vi "Initialize LMS Filter.vi"(0 "reference in":refnum<class "AdvSigProc.lvclass">, 5 "error in (no error)":errorcluster, 6 "Reset Filter?":bool=TRUE) -> (14 "reference out":refnum<class "AdvSigProc.lvclass">, 19 "error out":errorcluster)   [LabVIEW 2020, in "AdvSigProc.lvclass"]
uses:
  AdvSigProc.lvclass
  protected/Iteration Metrics.ctl
  <vilib>/addons/Adaptive Filters/Create/AFT Create FIR LMS (Real).vi
  <vilib>/addons/Adaptive Filters/Create/AFT Create FIR RLS (Real).vi
  <vilib>/addons/Adaptive Filters/Create/AFT Create FIR QR-RLS (Real).vi
  <vilib>/addons/Adaptive Filters/Create/AFT Create FIR Normalized LMS (Real).vi
  <vilib>/addons/Adaptive Filters/NI_AdaptiveFilter.lvlib
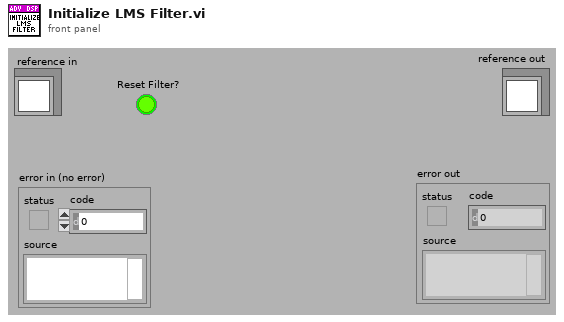
[diagram p1: front panel]
types:
  T1 = typedef "AdvSigProc.lvclass/Iteration Metrics.ctl" = cluster{"Name":string, "Max":dbl, "Min":dbl, "Values History":dbl[]}
  T2 = typedef "AdvSigProc.lvclass/ObjectAttributesRef.ctl" = refnum<data-value>
  T3 = typedef "AdvSigProc.lvclass/ObjectAttributes.ctl" = cluster{"Time Data":cluster{"New Time Data Obj?":bool, "GSwFormDSP":refnum<class "GSwFormDSP.lvclass">}, "LMS Parameters":T4}
  T4 = typedef "AdvSigProc.lvclass/LMS.ctl" = cluster{"adaptive filter Ref":refnum<k20>, "Filtered Signals":refnum<class "GSwFormDSP.lvclass">, "Filter Coefs":dbl[], "Input Parameters":T5, "Iteration Metrics":T1[]}
  T5 = typedef "AdvSigProc.lvclass/LMS Input Parameters.ctl" = cluster{"Type":enum16{"Normalized LMS", "LMS", "FIR Sign LMS", "FIR Fast Block LMS", "RLS", "QR - RLS"}, "Filter Class":enum16{"Noise Cancelling (BGN Ref)", "Noise Cancelling (Speech Ref)"}, "Filter Length":i32, "µ Parameters":cluster{"Type":enum16{"User Input", "Auto µ"}, "step size":dbl}, "Iterations":cluster{"Current":i32, "Maximum":i32}}
  T6 = enum16{"Normalized LMS", "LMS", "FIR Sign LMS", "FIR Fast Block LMS", "RLS", "QR - RLS"}
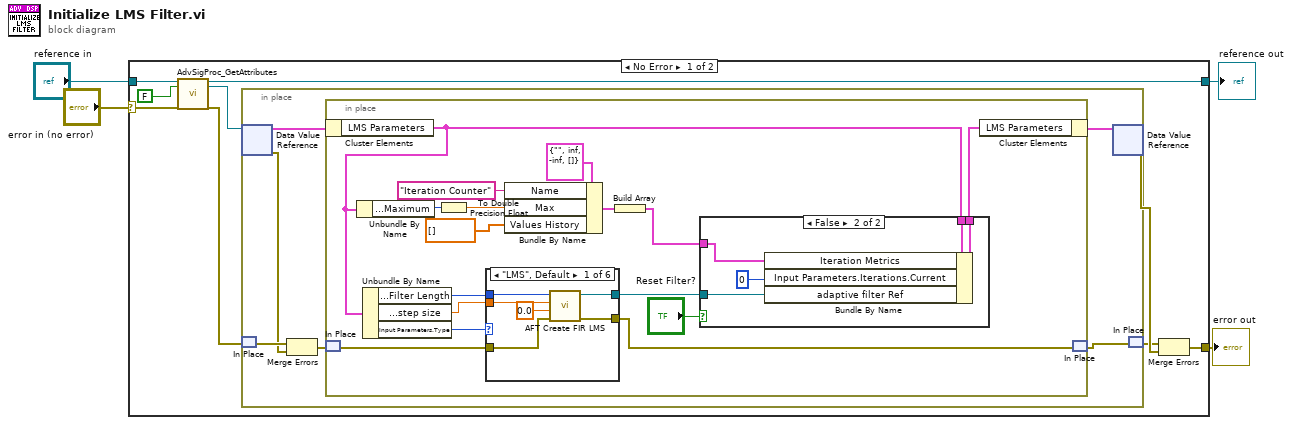
[diagram p0: block diagram]
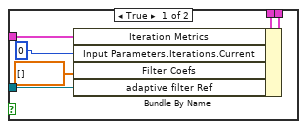
[diagram p2: hidden frame]
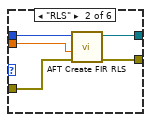
[diagram p3: hidden frame]
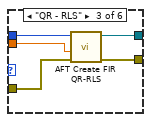
[diagram p4: hidden frame]
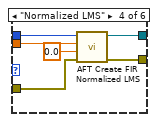
[diagram p5: hidden frame]
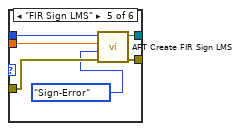
[diagram p6: hidden frame]
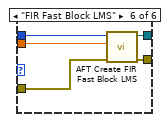
[diagram p7: hidden frame]
diagram:
  n1 = case shown="No Error" "error in (no error)" {
    selector: "error in (no error)" -> [w9 w81]
    tunnel: [w13 w81] -> w3
    tunnel: [w8 w80] -> w1
    tunnel: "reference in" -> [w11 w80]
    frame No Error {
      n2 = call "AdvSigProc_GetAttributes.vi"("reference in"=w11, "return data? (T)"=FALSE, "error in (no error)"=w9) -> ("reference out"=w8:refnum<class "AdvSigProc.lvclass">, "attributes ref"=w7:T2, "error out"=w6:errorcluster)  [unwired: 13 in, 1 out]
      n3 = in-place {
        n4 = in-place-dvr #1(w7) -> (w18:T3, w16:errorcluster)
        n5 = in-place-match #2(w6) -> (w17:errorcluster)
        n6 = Merge Errors(w17, w16) -> (w15:errorcluster)
        n7 = in-place {
          n8 = in-place-cluster #3(w18) -> ("LMS Parameters"=w26:T4)
          n9 = in-place-match #4(w15) -> (w31:errorcluster)
          n10 = Unbundle By Name(w26) -> ("Input Parameters.Iterations.Maximum"=w25:i32)
          n11 = Unbundle By Name(w26) -> ("Input Parameters.Filter Length"=w34:i32, "Input Parameters.µ Parameters.step size"=w33:dbl, "Input Parameters.Type"=w32:T6)
          n12 = To Double Precision Float(number=w25) -> (double precision float=w24:dbl)
          n13 = case shown="\"LMS\", Default" w32 {
            tunnel: w34 -> [w52 w57 w62 w68 w74 w79]
            tunnel: w33 -> [w50 w55 w61 w66 w73 w78]
            tunnel: w31 -> [w49 w56 w60 w65 w72 w77]
            tunnel: [w48 w53 w58 w64 w71 w76] -> w30
            tunnel: [w47 w54 w59 w63 w70 w75] -> w29
            frame "LMS", Default {
              n14 = call-poly <vilib>:"AFT Create FIR LMS.vi"("error in (no error)"=w49, "leakage"=0.0, "step size"=w50, "filter length"=w52) -> ("error out"=w47:errorcluster, "adaptive filter out"=w48:refnum<k20>)  [unwired: 6 in]
            }
            frame "RLS" {
              n15 = call-poly <vilib>:"AFT Create FIR RLS.vi"("error in (no error)"=w56, "regularization factor"=w55, "filter length"=w57) -> ("error out"=w54:errorcluster, "adaptive filter out"=w53:refnum<k20>)  [unwired: 7 in]
            }
            frame "QR - RLS" {
              n16 = call-poly <vilib>:"AFT Create FIR QR-RLS.vi"("error in (no error)"=w60, "regularization factor"=w61, "filter length"=w62) -> ("error out"=w59:errorcluster, "adaptive filter out"=w58:refnum<k20>)  [unwired: 7 in]
            }
            frame "Normalized LMS" {
              n17 = call-poly <vilib>:"AFT Create FIR Normalized LMS.vi"("error in (no error)"=w65, "leakage"=0.0, "step size"=w66, "filter length"=w68) -> ("error out"=w63:errorcluster, "adaptive filter out"=w64:refnum<k20>)  [unwired: 6 in]
            }
            frame "FIR Sign LMS" {
              n18 = call <vilib>:"AFT Create FIR Sign LMS.vi"("error in (no error)"=w72, "sign type"=enum16{"Sign-Error", "Sign-Data", "Sign-Sign"}."Sign-Error", "step size"=w73, "filter length"=w74) -> ("error out"=w70:errorcluster, "adaptive filter out"=w71:refnum<k20>)  [unwired: 6 in]
            }
            frame "FIR Fast Block LMS" {
              n19 = call <vilib>:"AFT Create FIR Fast Block LMS.vi"("error in (no error)"=w77, "step size"=w78, "filter length"=w79) -> ("error out"=w75:errorcluster, "adaptive filter out"=w76:refnum<k20>)  [unwired: 7 in]
            }
          }
          n20 = Bundle By Name(cluster=T1 {"Name"="", "Max"=inf, "Min"=-inf, "Values History"=[]} ("Iteration Metric"), "Name"="Iteration Counter", "Max"=w24, "Values History"=dbl[] [] ("Filter Coefs")) -> (w21:T1)
          n21 = Build Array(w21) -> (w20:T1[])
          n22 = case shown="False" "Reset Filter?" {
            tunnel: [w41 w46] -> w35
            tunnel: w26 -> [w40 w45]
            tunnel: w30 -> [w39 w44]
            tunnel: w20 -> [w36 w42]
            frame True {
              n23 = Bundle By Name(cluster=w40, "Iteration Metrics"=w36, "Input Parameters.Iterations.Current"=0 ("Iterations.Current"), "Filter Coefs"=dbl[] [], "adaptive filter Ref"=w39) -> (w41:T4)
            }
            frame False {
              n24 = Bundle By Name(cluster=w45, "Iteration Metrics"=w42, "Input Parameters.Iterations.Current"=0 ("Iterations.Current"), "adaptive filter Ref"=w44) -> (w46:T4)
            }
          }
          n25 = in-place-cluster #3("LMS Parameters"=w35) -> (w19:T3)
          n26 = in-place-match #4(w29) -> (w14:errorcluster)
        }
        n27 = in-place-dvr #1(w19) -> (w12:errorcluster)  [unwired: 1 out]
        n28 = in-place-match #2(w14) -> (w5:errorcluster)
      }
      n29 = Merge Errors(w5, w12) -> (w13:errorcluster)
    }
    frame Error {
    }
  }
  "error out" <- w3
  "reference out" <- w1
